vi "Set Run Control.vi"(8 "error in (no error)":errorcluster, 10 "Run Control":T1, 11 "PicoScope 3000a in":refnum<class "PicoScope 3000a.lvclass">) -> (0 "error out":errorcluster, 3 "PicoScope 3000a out":refnum<class "PicoScope 3000a.lvclass">)   [LabVIEW 2018, in "PicoScope 3000a.lvlib" / "PicoScope 3000a.lvclass"]
doc: "This Override method is used to set the Oscope instrument running mode. The 'Run Control' control has 3 modes of operation: 0-Run (or continuous), 1 - Single, 2 - Stop."
uses:
  PicoScope 3000a.lvclass
  PPLs/Oscilloscope/Parent/Oscilloscope.lvlibp/Custom Controls/Run Control.ctl
  PPLs/Oscilloscope/Parent/Oscilloscope.lvlibp
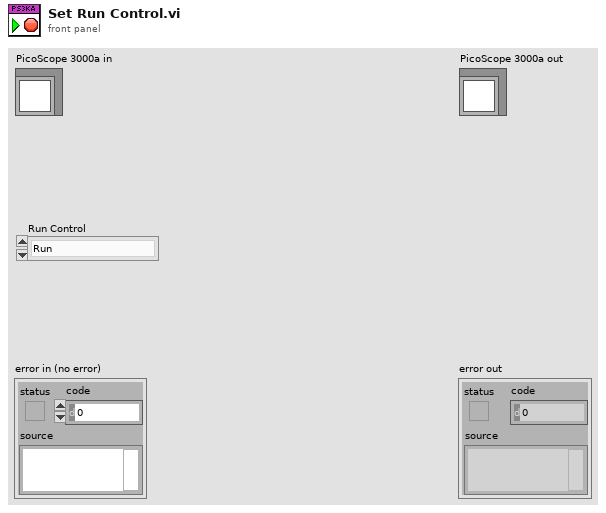
[diagram p1: front panel]
types:
  T1 = typedef "Oscilloscope.lvlibp/Run Control.ctl" = enum16{"Run", "Single", "Stop"}
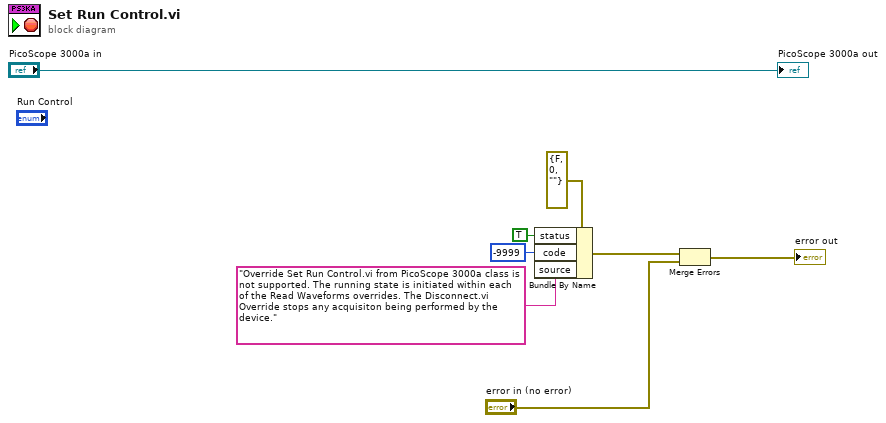
[diagram p0: block diagram]
diagram:
  n1 = Bundle By Name(cluster=errorcluster {"status"=FALSE, "code"=0, "source"=""} ("error constant"), "status"=TRUE, "code"=-9999, "source"="Override Set Run Control.vi from PicoScope 3000a class is not supported. The running state is initiated within each of the Read Waveforms overrides. The Disconnect.vi Override stops any acquisiton being performed by the device.") -> (w4:errorcluster)
  n2 = Merge Errors(w4, "error in (no error)") -> (→"error out":errorcluster)
  "PicoScope 3000a out" <- "PicoScope 3000a in"
